vi "Get Configuration.vi"(7 "Plugin Name":string, 8 "error in (no error)":errorcluster, 10 "Index":i32, 11 "CIF_Plugin_UI in":refnum<class "CIF_Plugin_UI.lvclass">) -> (0 "error out":errorcluster, 1 "Not Found":bool, 2 "JSON Configuration":string, 3 "CIF_Plugin_UI out":refnum<class "CIF_Plugin_UI.lvclass">)   [LabVIEW 2021, in "CIF_Plugin_UI.lvclass"]
uses:
  CIF_Plugin_UI.lvclass
  D:/dev/CIF-LVCore/src/CIFUI/CIF_UI.lvclass
  CIFUI/CIF_UI.lvclass
  CIFCore/Grpc/CIFCoreWrapper/CIFCoreWrapper.lvlib
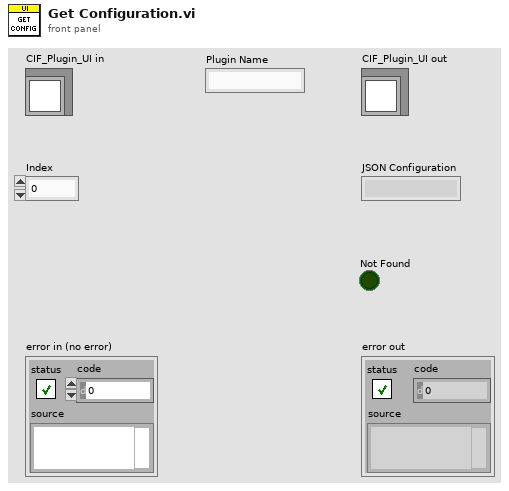
[diagram p1: front panel]
types:
  T1 = typedef "grpc-lvsupport-release.lvlib/grpcId.ctl" = u64
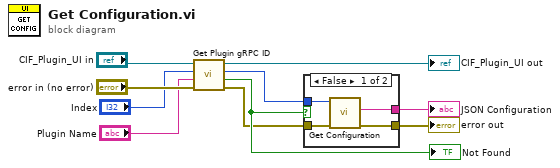
[diagram p0: block diagram]
diagram:
  n1 = call "Get Plugin gRPC ID.vi"("error in (no error)"="error in (no error)", "Plugin Name"="Plugin Name", "Index"="Index", "CIF_UI in"="CIF_Plugin_UI in") -> ("error out"=w4:errorcluster, "Not Found"=w5:bool, "gRPC ID"=w6:T1, "CIF_UI out"=→"CIF_Plugin_UI out":refnum<class "CIF_Plugin_UI.lvclass">)  [unwired: 4 in]
  "Not Found" <- w5
  n2 = case shown="False" w5 {
    tunnel: w6 -> [w14 _]
    tunnel: w4 -> [w13 w15]
    tunnel: [w12 w15] -> w3
    tunnel: [w11 _] -> w1
    frame False {
      n3 = call "Get Configuration.vi"("error in"=w13, "gRPC ID"=w14) -> ("error out"=w12:errorcluster, "JSON Configuration"=w11:string)  [unwired: 7 in, 1 out]
    }
    frame True {
    }
  }
  "error out" <- w3
  "JSON Configuration" <- w1
